vi "thermo_status2string.vi"(5 "to upper case":bool, 7 "add channel":bool, 8 "prefix":string, 9 "thermo":T1={"stat"=enum."Disabled", "type"=enum."COMET Tx5xx (ethernet)", "comment"="", "tag"="", "refresh"=5.0, "IP"="192.168.2.34", "port"=502, "VISA"="", "last readout"=timestamp(0 s since 1904-01-01), "TCP ref"=refnum, "VISA sess"="", "idn"="", "press"=0.0, "RH"=0.0, "temp"=0.0, "pres cor"=[], "RH cor"=[], "temp cor"=[], "try left"=0, "failed"=FALSE, "RTD set"=[], "RTD inv"=[], "range"=0.0, "net mode"=enum."MODBUS"} {"RTD inv" format="%.1f"; "RTD set" format="%.1f"; "temp cor" format="%.1f"; "RH cor" format="%.1f"; "pres cor" format="%.1f"; "refresh" min=0.1 max=1000.0 format="%.2f"}, 10 "index":u8, 11 "status code":i32) -> (0 "message available":bool, 3 "status string":string)   [LabVIEW 2013]
uses:
  thermo.ctl
  thermo_types.ctl
  thermo_var.vi
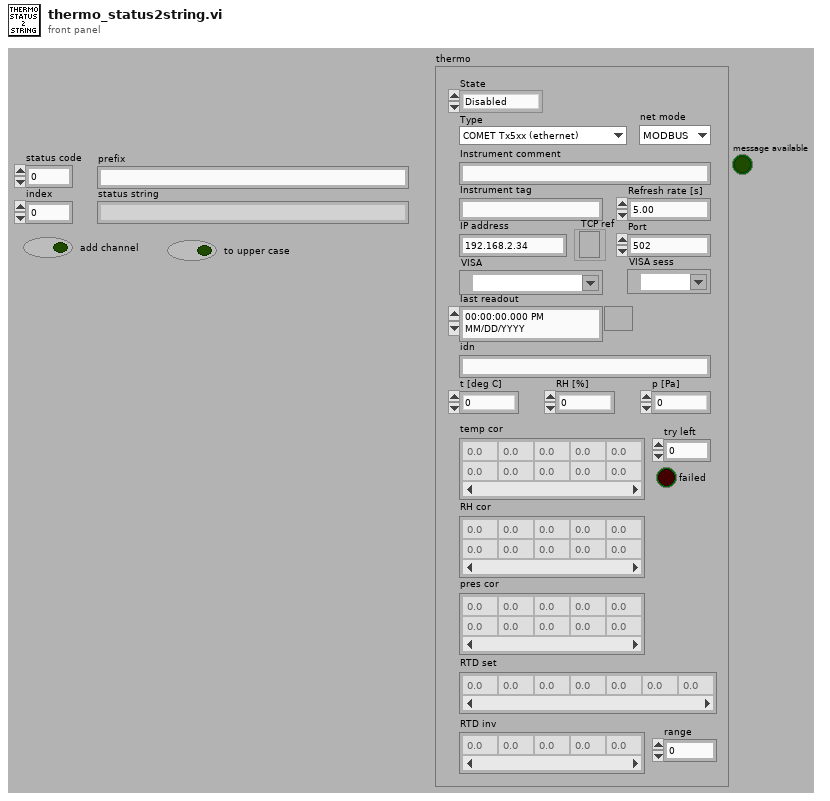
[diagram p1: front panel]
types:
  T1 = typedef "thermo.ctl" = cluster{"stat":enum16{"Disabled", "Enabled"}, "type":T2, "comment":string, "tag":string, "refresh":dbl, "IP":string, "port":u16, "VISA":refnum<visa-resource-name>, "last readout":timestamp, "TCP ref":refnum<k5>, "VISA sess":refnum<visa-resource-name>, "idn":string, "press":dbl, "RH":dbl, "temp":dbl, "pres cor":dbl[][], "RH cor":dbl[][], "temp cor":dbl[][], "try left":i32, "failed":bool, "RTD set":dbl[], "RTD inv":dbl[], "range":dbl, "net mode":enum16{"MODBUS", "HTTP"}}
  T2 = typedef "thermo_types.ctl" = enum16{"COMET Tx5xx (ethernet)", "Keithley 2002 (GPIB) + RTD", "Agilent 344xx (GPIB) + RTD"}
  T3 = enum16{"Stop trying - keep last value", "Stop trying - return zeroes", "Generate error - stop sweep"}
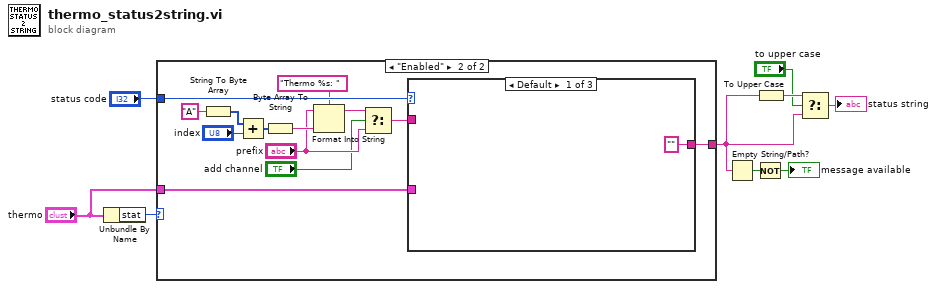
[diagram p0: block diagram]
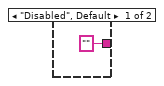
[diagram p2: hidden frame]
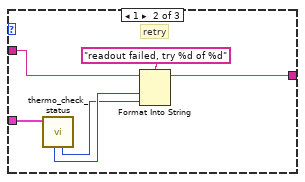
[diagram p3: hidden frame]
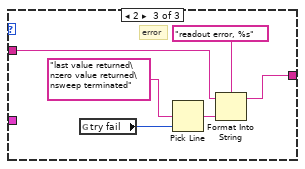
[diagram p4: hidden frame]
diagram:
  n1 = Unbundle By Name("thermo") -> ("stat"=w9:enum16{"Disabled", "Enabled"})
  n2 = case shown="\"Enabled\"" w9 {
    tunnel: "status code" -> [_ w23]
    tunnel: "thermo" -> [_ w12]
    tunnel: ["" w11] -> w3
    frame "Disabled", Default {
    }
    frame "Enabled" {
      n3 = String To Byte Array(string="A") -> (unsigned byte array=w20:u8[])
      n4 = Add(x=w20, y="index") -> (x+y=w19:u8[])
      n5 = Byte Array To String(unsigned byte array=w19) -> (string=w18:string)
      n6 = Format Into String(format string="Thermo %s: ", initial string="prefix", w18) -> (resulting string=w16:string)  [unwired: 1 in, 1 out]
      n7 = Select(t=w16, s="add channel", f="prefix") -> (s? t:f=w13:string)
      n8 = case shown="Default" w23 {
        tunnel: w13 -> [_ w30 w35]
        tunnel: w12 -> [_ w28 _]
        tunnel: ["" w25 w36] -> w11
        frame Default {
        }
        frame 1 {
          # "retry"
          n9 = call "thermo_check_status.vi"("channel"=w28) -> ("retry N"=w26:i32, "try"=w27:i32)  [unwired: 5 in, 4 out]
          n10 = Format Into String(format string="readout failed, try %d of %d", initial string=w30, w27, w26) -> (resulting string=w25:string)  [unwired: 1 in, 1 out]
        }
        frame 2 {
          # "error"
          n11 = global read "thermo_var.vi" "try fail"() -> (w32:T3)
          n12 = Pick Line(multi-line string="last value returned\nzero value returned\nsweep terminated" ("string (\"\")"), line index=w32) -> (output string=w34:string)  [unwired: 1 in]
          n13 = Format Into String(format string="readout error, %s", initial string=w35, w34) -> (resulting string=w36:string)  [unwired: 1 in, 1 out]
        }
      }
    }
  }
  n14 = Empty String/Path?(string/path=w3) -> (empty?=w6:bool)
  n15 = Not(x=w6) -> (.not. x?=→"message available":bool)
  n16 = To Upper Case(1:w3) -> (0:w4:string)
  n17 = Select(t=w4, s="to upper case", f=w3) -> (s? t:f=→"status string":string)
